vi "PH_Cont-601k_PSU.Action Set Configuration.vi"(0 "VI in":refnum<vi>, 2 "Configuration":T1 items=["Ch intl, Fl intl, QSw intl", "Ch intl, Fl intl, QSw ext", "Ch intl, Fl ext, QSw intl", "Ch intl, Fl ext, QSw ext", "Ch ext, Fl int, QSw int", "Ch ext, Fl int, QSw ext", "Ch ext, Fl ext, QSw int", "Ch ext, Fl ext, QSw ext"], 5 "error in (no error)":errorcluster) -> (14 "VI out":refnum<vi>, 19 "error out":errorcluster)   [LabVIEW 2014, in "PH_Cont-601k_PSU.lvlib"]
uses:
  PH_Cont-601k_PSU.lvlib
  PH_Cont-601k_PSU.Configuration.ctl
  PH_Cont-601k_PSU.Readyness Device.ctl
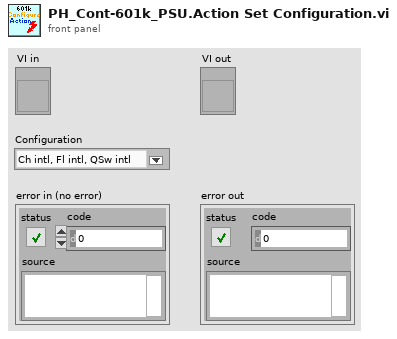
[diagram p1: front panel]
types:
  T1 = typedef "PH_Cont-601k_PSU.lvlib/PH_Cont-601k_PSU.Configuration.ctl" = u16
  T2 = typedef "PH_Cont-601k_PSU.lvlib/PH_Cont-601k_PSU.Readyness Device.ctl" = enum32{"OFF", "CONNECTING", "CONNECTED", "OPERATING", "EOC", "ERROR"}
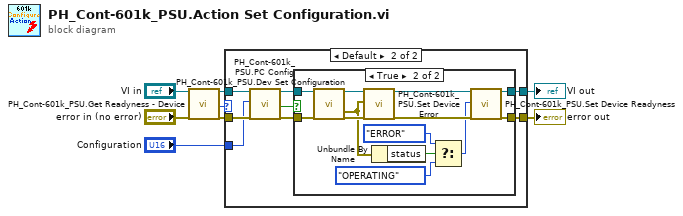
[diagram p0: block diagram]
diagram:
  n1 = call "PH_Cont-601k_PSU.Get Readyness - Device.vi"("VI in"="VI in", "error in (no error)"="error in (no error)") -> ("VI out"=w4:refnum<vi>, "Readyness - Device"=w7:T2, "error out"=w6:errorcluster)  [unwired: 15 in]
  n2 = case shown="Default" w7 {
    tunnel: w6 -> [w9 w18]
    tunnel: [w9 w17] -> w1
    tunnel: w4 -> [w10 w16]
    tunnel: [w10 w15] -> w2
    tunnel: "Configuration" -> [_ w11]
    frame "OFF" {
    }
    frame Default {
      n3 = call "PH_Cont-601k_PSU.PC Config.vi"("VI in"=w16, "Configuration"=w11, "error in (no error)"=w18) -> ("VI out"=w14:refnum<vi>, "\"Config\" changed"=w12:bool, "error out"=w13:errorcluster)  [unwired: 14 in]
      n4 = case shown="True" w12 {
        tunnel: [w19 w21] -> w17
        tunnel: [w20 w22] -> w15
        tunnel: w14 -> [w20 w33]
        tunnel: w13 -> [w19 w32]
        frame False {
        }
        frame True {
          n5 = call "PH_Cont-601k_PSU.Dev Set Configuration.vi"("VI in"=w33, "error in (no error)"=w32) -> ("VI out"=w25:refnum<vi>, "Device Error out"=w23:errorcluster, "error out"=w24:errorcluster)  [unwired: 15 in]
          n6 = call "PH_Cont-601k_PSU.Set Device Error.vi"("VI in"=w25, "Device Error"=w23, "error in (no error)"=w24) -> ("VI out"=w30:refnum<vi>, "error out"=w31:errorcluster)  [unwired: 15 in]
          n7 = Unbundle By Name(w23) -> ("status"=w27:bool)
          n8 = Select(t=PH_Cont-601k_PSU.Readyness_Device."ERROR" ("Readyness.Device"), s=w27, f=PH_Cont-601k_PSU.Readyness_Device."OPERATING" ("Readyness Device to set")) -> (s? t:f=w29:T2)
          n9 = call "PH_Cont-601k_PSU.Set Device Readyness.vi"("VI in"=w30, "Readyness Device to set"=w29, "error in (no error)"=w31) -> ("VI out"=w22:refnum<vi>, "error out"=w21:errorcluster)  [unwired: 15 in]
        }
      }
    }
  }
  "VI out" <- w2
  "error out" <- w1
